vi "Power Interface Detector.vi"(1 "Power interface finder Loop ID":u16, 11 "error in (no error)":errorcluster) -> ()   [LabVIEW 2011]
uses:
  Magna Interface/Magna Commands.ctl
  Application Structure/Loop ID.ctl
  emi Lib/System 01/0 - General/App/Loop control 2/Private/_emi_SMLoop Control Single.vi
  emi Lib/System 01/0 - General/App/Loop control 2/Private/_emi_ SMLoop start condition.vi
  emi Lib/System 01/0 - General/App/Loop control 2/Private/_emi_ SMLoop Error Check.vi
  emi Lib/Basic/0 - General/Error/emi_Is Error.vi
  emi Lib/System 01/0 - General/App/Loop control 2/Private/_emi_SMLoop Register new.vi
  emi Lib/System 01/0 - General/S&E reporting/emi_Send S&E Error message.vi
  emi Lib/Basic/0 - General/Error/emi_ Is Error state.vi
  emi Lib/System 01/0 - General/emi_Read System ID.vi
  emi Lib/System 01/0 - General/App/Loop control/Private/_emi_GFV Loop Linking.vi
  emi Lib/System 01/0 - General/App/Loop control/Private/_emi_GFV Loop Enable.vi
  emi Lib/System 01/0 - General/App/Loop control 2/Private/_emi_ SMLoop Restart.vi
  emi Lib/System 01/0 - General/App/Private/_emi_GFV App Close.vi
  emi Lib/System 01/0 - General/App/Loop control 2/Private/_emi_ SMLoop Restart Counter.vi
  emi Lib/System 01/0 - General/App/Loop control/Private/_emi_GFV Loop Running.vi
  emi Lib/System 01/0 - General/Private/_emi_GFV System ID.vi
  emi Lib/System 01/0 - General/S&E reporting/Private/_emi_S&E Q Generator.vi
  emi Lib/System 01/0 - General/App/Loop control/Private/_emi_GFV stop a loop so it can reset.vi
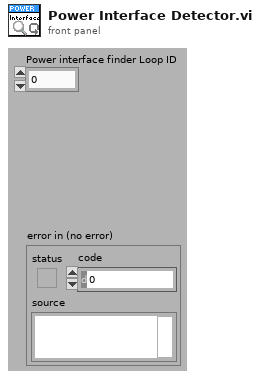
[diagram p1: front panel]
types:
  T1 = typedef "Magna Commands.ctl" = enum16{"Read Inputs", "HV ON", "HV OFF", "Set Resistance", "Set Head Voltage SP"}
  T2 = typedef "Loop ID.ctl" = enum16{"Main-QSM", "Main-Dialog", "Main-Ind Upd", "Main-Graph Upd", "Main-Debug", "Main-DebugW1", "Main-DebugW2", "Main-SE Handler", "Interface-PCP", "Interface-CANbus", "Interface-Modem", "Var Handling-Beat", "Var Handling-From PCP", "Var Handling-File storage", "Var Handling-From Simulator", "GUI-GrphW Mast", "GUI-GrphW Slav", "SIM-Tool W1", "SIM-Tool W2", "Alm-Sound", "LEIN-motor", "Tool data gatherer Qer", "Tool Data LEIN STAT2 dekoder", "Indicator Value Update", "Tool STAT2 dedicated reader", "Tool ID handler", "Detail View L1", "Detail View L2", "Main display enable view", "Sequence runner", "Voltage setpoint", "Resistance setpoint", "Stroker Wizard L1", "Stroker Wizard L2", "Alarm Handling", "Annotations Tip Strip", "Magna Interface", "Modem Status", "Var Handling - Modem Status", "Power interface detector"}
  T3 = typedef "_emi_ SMLoop sates.ctl" = enum16{"Init", "Standby", "Start", "Normal Operation", "Stop", "Error Handling", "End", "Post"}
  T4 = cluster{"Placeholder":bool, "VISA name":refnum<visa-resource-name>}
  T5 = typedef "PSU Type.ctl" = enum16{"Unipower", "Magna 8.3A", "Magna 12A", "None"}
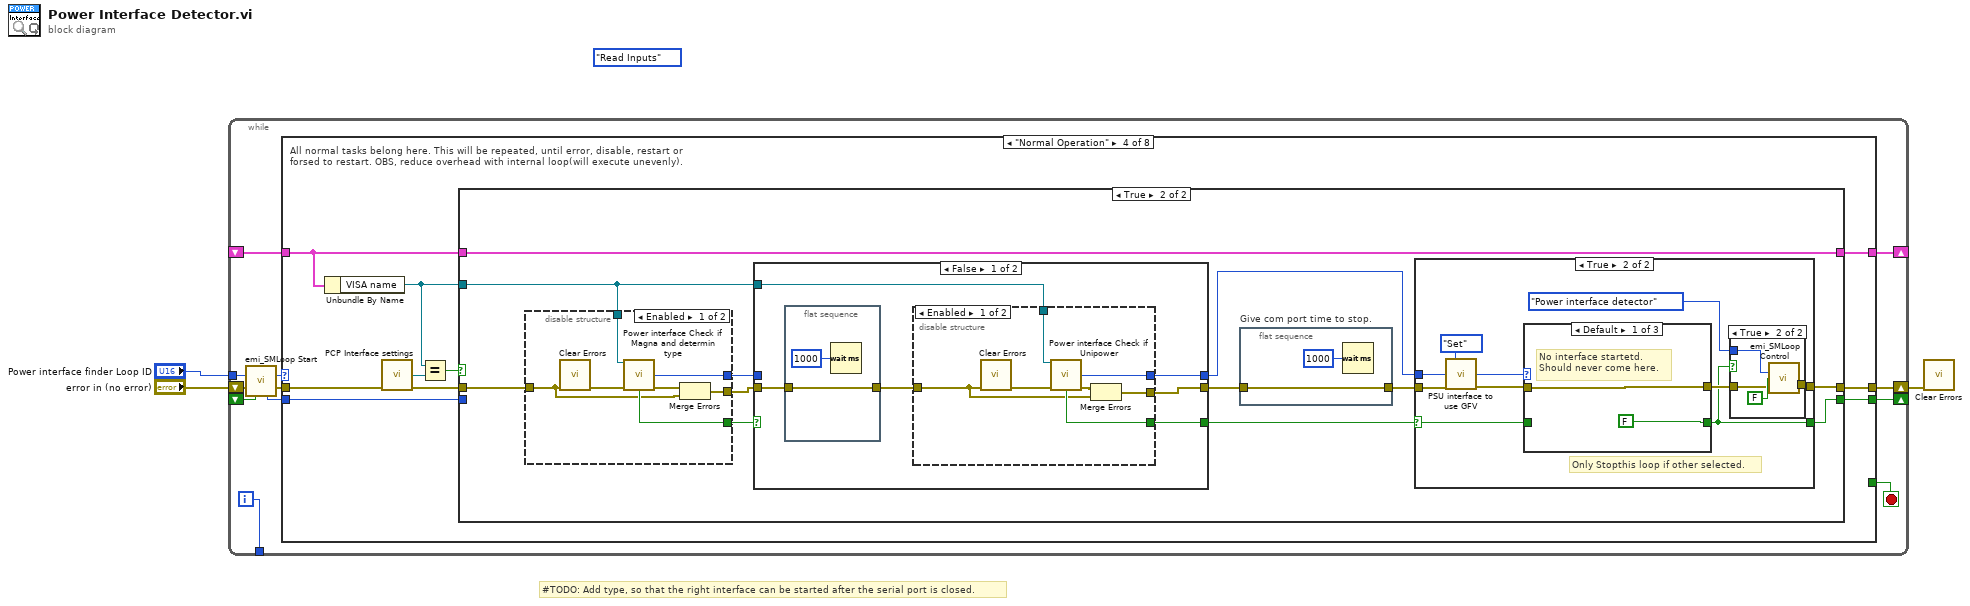
[diagram p0: block diagram]
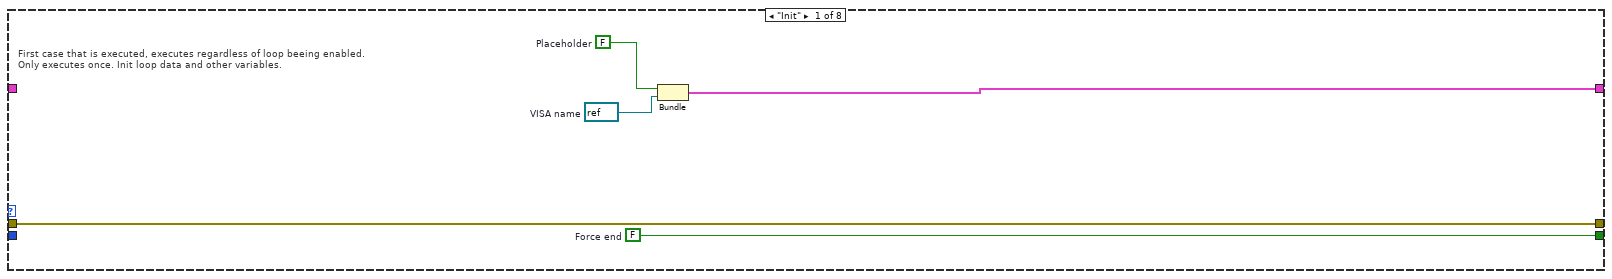
[diagram p2: hidden frame]
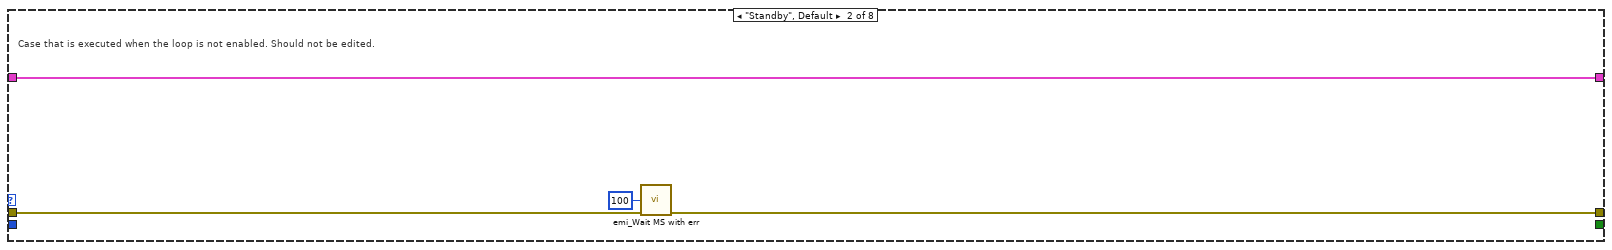
[diagram p3: hidden frame]
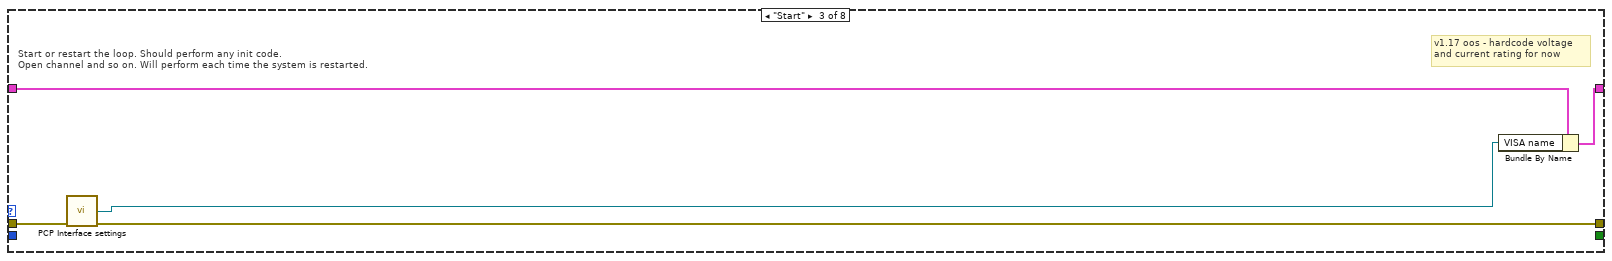
[diagram p4: hidden frame]
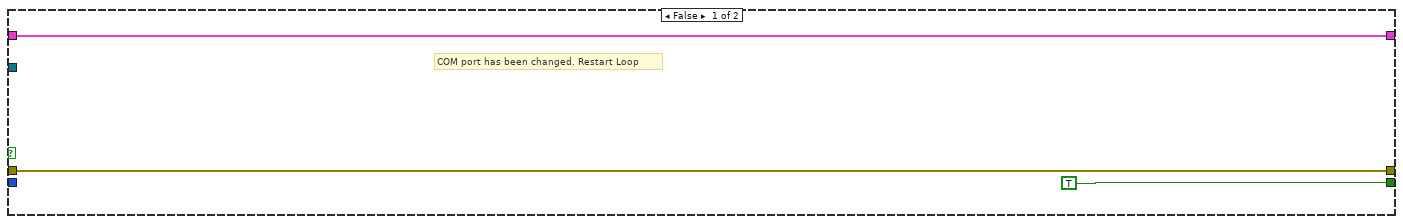
[diagram p5: hidden frame]
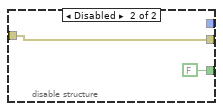
[diagram p6: hidden frame]
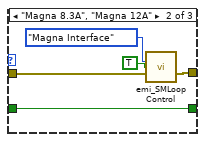
[diagram p9: hidden frame]
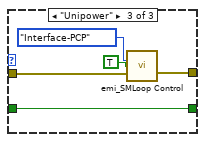
[diagram p10: hidden frame]
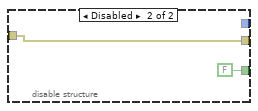
[diagram p11: hidden frame]
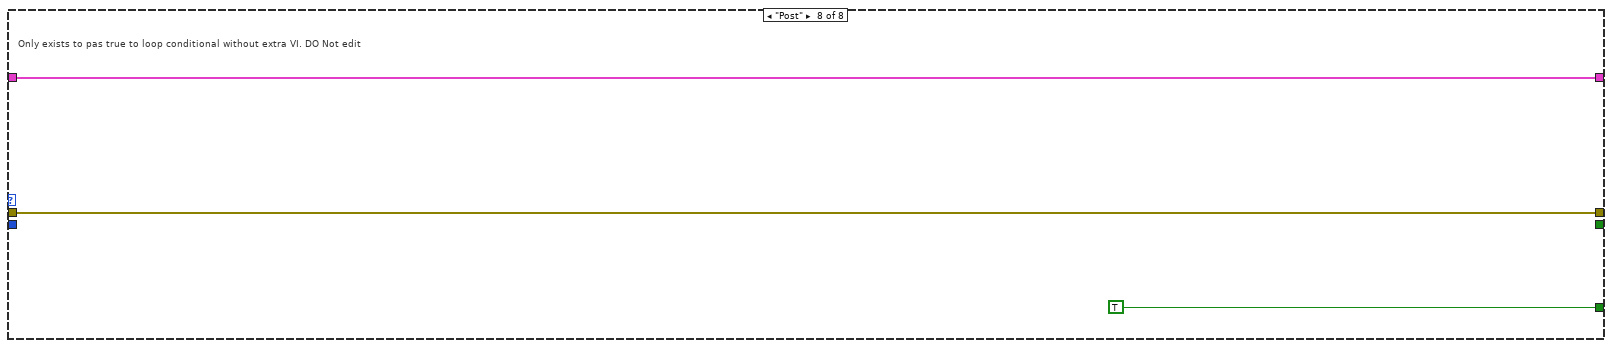
[diagram p16: hidden frame]
diagram:
  (unwired) Magna_Commands."Read Inputs" ("Action")
  # "#TODO: Add type, so that the right interface can be started after the serial port is closed."
  n1 = while {
    shift-right: [w15] -> _
    shift-left: _ -> [w11]
    shift-right: [w13] -> w1
    shift-left: "error in (no error)" -> [w9]
    tunnel: [w12] -> _
    shift-right: [w10] -> _
    shift-left: _ -> [w5]
    tunnel: "Power interface finder Loop ID" -> [w6]
    i -> [w12]
    stop <- w14 stop-if-true
    n2 = call "emi_SMLoop Start.vi"("Loop ID"=w6, "error in (no error)"=w9, "Force Stop(F)"=w5) -> ("Loop command"=w7:T3, "error out"=w8:errorcluster, "Loop ID out"=w4:i32)  [unwired: 10 in]
    n3 = case shown="\"Normal Operation\"" w7 {
      tunnel: [w18 w21 w28 w37 w116 w118 w119 w122] -> w15
      tunnel: [_ _ _ _ _ _ _ TRUE] -> w14
      tunnel: w8 -> [w16 w23 w29 w39 w115 w117 w120 w123]
      tunnel: [w16 w22 w25 w38 w115 w117 w120 w123] -> w13
      tunnel: w11 -> [_ w21 w27 w36 w116 w118 w119 w122]
      tunnel: [w19 _ _ w35 _ _ _ _] -> w10
      tunnel: w4 -> [_ _ _ w34 _ _ _ _]
      frame "Init" {
        w17 = refnum<visa-resource-name> refnum  # VISA name
        w19 = FALSE  # Force end
        w20 = FALSE  # Placeholder
        # "First case that is executed, executes regardless of loop beeing enabled.\nOnly executes once. Init loop data and other variables."
        n4 = Bundle("Placeholder"=w20, "VISA name"=w17) -> (w18:T4)  [unwired: 1 in]
      }
      frame "Standby", Default {
        # "Case that is executed when the loop is not enabled. Should not be edited."
        n5 = call "emi_Wait MS with err.vi"("milliseconds to wait(0)"=u32 100, "error in (no error)"=w23) -> ("error out"=w22:errorcluster)  [unwired: 13 in]
      }
      frame "Start" {
        # "v1.17 oos - hardcode voltage \nand current rating for now"
        # "Start or restart the loop. Should perform any init code. \nOpen channel and so on. Will perform each time the system is restarted."
        n6 = call "PCP Interface settings.vi"("error in (no error)"=w29) -> ("PCP VISA  name  out"=w26:refnum<visa-resource-name>, "error out"=w25:errorcluster)  [unwired: 13 in]
        n7 = Bundle By Name(cluster=w27, "VISA name"=w26) -> (w28:T4)
      }
      frame "Normal Operation" {
        # "All normal tasks belong here. This will be repeated, until error, disable, restart or\nforsed to restart. OBS, reduce overhead with internal loop(will execute unevenly)."
        n8 = Unbundle By Name(w36) -> ("VISA name"=w30:refnum<visa-resource-name>)
        n9 = call "PCP Interface settings.vi"("error in (no error)"=w39) -> ("PCP VISA  name  out"=w33:refnum<visa-resource-name>, "error out"=w31:errorcluster)  [unwired: 13 in]
        n10 = Equal?(x=w30, y=w33) -> (x = y?=w32:bool)
        n11 = case shown="True" w32 {
          tunnel: w31 -> [w41 w50]
          tunnel: [w40 w54] -> w37
          tunnel: w36 -> [w40 w54]
          tunnel: [TRUE ("Force End") w48] -> w35
          tunnel: [w41 w46] -> w38
          tunnel: w30 -> [_ w53]
          tunnel: w34 -> [_ _]
          frame False {
            # "COM port has been changed. Restart Loop"
          }
          frame True {
            n12 = disable-structure shown="Enabled" {
              disable-tunnel: w53 -> [w61 _]
              disable-tunnel: [w60 FALSE ("Found PSU")] -> w52
              disable-tunnel: [w59 _] -> w51
              disable-tunnel: w50 -> [w56 w63]
              disable-tunnel: [w55 w63] -> w49
              frame Enabled {
                n13 = call <vilib>:"Clear Errors.vi"("error in (no error)"=w56) -> ("error out"=w58:errorcluster)  [unwired: 6 in]
                n14 = call "Power interface Check if Magna and determin type.vi"("VISA Refnum in"=w61, "error in (no error)"=w58) -> ("PSU type"=w59:T5, "Found PSU"=w60:bool, "error out"=w57:errorcluster)  [unwired: 11 in]
                n15 = Merge Errors(w57, w56) -> (w55:errorcluster)
              }
              frame Disabled {
              }
            }
            n16 = case shown="False" w52 {
              selector: w52 -> [_ w114]
              tunnel: w49 -> [w97 w112]
              tunnel: w53 -> [w100 _]
              tunnel: w51 -> [_ w113]
              tunnel: [w96 w112] -> w44
              tunnel: [w98 w114] -> w47
              tunnel: [w99 w113] -> w45
              frame False {
                n17 = flat-sequence {
                  tunnel: [w111] -> w95
                  tunnel: w97 -> [w111]
                  frame #0 {
                    n18 = Wait (ms)(milliseconds to wait=u32 1000) -> ()  [unwired: 1 out]
                  }
                }
                n19 = disable-structure shown="Enabled" {
                  disable-tunnel: w100 -> [w107 _]
                  disable-tunnel: [w105 _] -> w99
                  disable-tunnel: [w104 FALSE ("Found PSU")] -> w98
                  disable-tunnel: [w103 w109] -> w96
                  disable-tunnel: w95 -> [w101 w109]
                  frame Enabled {
                    n20 = call <vilib>:"Clear Errors.vi"("error in (no error)"=w101) -> ("error out"=w102:errorcluster)  [unwired: 6 in]
                    n21 = call "Power interface Check if Unipower.vi"("VISA Refnum in"=w107, "error in (no error)"=w102) -> ("PSU type"=w105:T5, "Found PSU"=w104:bool, "error out"=w106:errorcluster)  [unwired: 11 in]
                    n22 = Merge Errors(w106, w101) -> (w103:errorcluster)
                  }
                  frame Disabled {
                  }
                }
              }
              frame True {
                # "Magna found"
              }
            }
            n23 = flat-sequence "Give com port time to stop." {
              tunnel: [w65] -> w43
              tunnel: w44 -> [w65]
              frame #0 {
                n24 = Wait (ms)(milliseconds to wait=u32 1000) -> ()  [unwired: 1 out]
              }
            }
            n25 = case shown="True" w47 {
              selector: w47 -> [w67 w72]
              tunnel: [w66 w69] -> w46
              tunnel: w43 -> [w66 w76]
              tunnel: [w67 w68] -> w48
              tunnel: w45 -> [_ w74]
              frame False {
                # "Not found. repeat the process"
              }
              frame True {
                # "Only Stopthis loop if other selected."
                n26 = call "PSU interface to use GFV.vi"("Action"=enum16{"Get", "Set"}."Set", "PSU type Inn in"=w74, "error in (no error)"=w76) -> ("PSU type  out"=w73:T5, "error out"=w75:errorcluster)  [unwired: 11 in]
                n27 = case shown="Default" w73 {
                  tunnel: [w84 w86 w91] -> w70
                  tunnel: w75 -> [w84 w87 w92]
                  tunnel: [FALSE w85 w90] -> w68
                  tunnel: w72 -> [_ w85 w90]
                  frame Default {
                    # "No interface startetd. \nShould never come here."
                  }
                  frame "Magna 8.3A", "Magna 12A" {
                    n28 = call-poly "emi_SMLoop Control.vi"("Loop ID in"=Loop_ID."Magna Interface" ("Loop ID"), "Enable"=TRUE, "error in (no error)"=w87) -> ("error out"=w86:errorcluster)  [unwired: 11 in, 1 out]
                  }
                  frame "Unipower" {
                    n29 = call-poly "emi_SMLoop Control.vi"("Loop ID in"=Loop_ID."Interface-PCP" ("Loop ID"), "Enable"=TRUE, "error in (no error)"=w92) -> ("error out"=w91:errorcluster)  [unwired: 11 in, 1 out]
                  }
                }
                n30 = case shown="True" w68 {
                  tunnel: Loop_ID."Power interface detector" ("Loop ID") -> [_ w79]
                  tunnel: w70 -> [w78 w81]
                  tunnel: [w78 w80] -> w69
                  frame False {
                  }
                  frame True {
                    n31 = call-poly "emi_SMLoop Control.vi"("Loop ID in"=w79, "Enable"=FALSE, "error in (no error)"=w81) -> ("error out"=w80:errorcluster)  [unwired: 11 in, 1 out]
                  }
                }
              }
            }
          }
        }
      }
      frame "Stop" {
        # "Stop the loop. May be restarted later. Close interfaces and the like"
      }
      frame "Error Handling" {
        # "Loop automaticaly returns here after error is found. If error is cleared, \nLoop wil continue as normal(if was operative when error."
      }
      frame "End" {
        # "Only executes at application end has. Should performa any action the loop \nneeds to finnish. Executes only once."
      }
      frame "Post" {
        # "Only exists to pas true to loop conditional without extra VI. DO Not edit"
      }
    }
  }
  n32 = call <vilib>:"Clear Errors.vi"("error in (no error)"=w1) -> ()  [unwired: 6 in, 1 out]
